vi "DefaultImageData.vi"() -> ()   [LabVIEW 2013, in "AnimatorXControl.xctl"]
uses:
  AnimatorXControl.xctl
  <vilib>/picture/picture.llb/imagedata.ctl
panel:
  out "DefaultImage":T1={"image type"=0, "image depth"=24, "image"=array[49152 elements], "mask"=[], "colors"=[], "Rectangle"={"left"=0, "top"=0, "right"=128, "bottom"=128}}
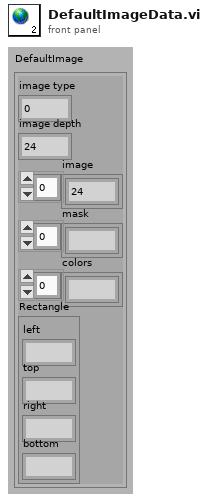
[diagram p1: front panel]
types:
  T1 = typedef "imagedata.ctl" = cluster{"image type":i32, "image depth":i32, "image":u8[], "mask":u8[], "colors":u32[], "Rectangle":cluster{"left":i16, "top":i16, "right":i16, "bottom":i16}}
diagram:
